vi "SetTemperatureSetPoint.vi"(2 "Temperature":sgl) -> ()   [LabVIEW 2011]
uses:
  GlobalVariables.vi
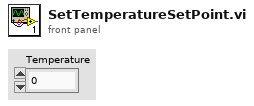
[diagram p1: front panel]
types:
  T1 = typedef "EZ-ZONE Output Cluster.ctl" = cluster{"Loop Control Mode":u32, "Closed Loop Set Point":sgl, "Open Loop Set Point":sgl, "Alarm 1 - High Set Point":sgl, "Alarm 1 - Low Set Point":sgl, "Alarm 2 - High Set Point":sgl, "Alarm 2 - Low Set Point":sgl, "Alarm 3 - High Set Point":sgl, "Alarm 3 - Low Set Point":sgl, "Alarm 4 - High Set Point":sgl, "Alarm 4 - Low Set Point":sgl, "Profile Action Request":u32, "Profile Start":u32, "Heat Proportional Band":sgl, "Cool Proportional Band":sgl, "Time Integral":sgl, "Time Derivative":sgl, "Heat Hysteresis":sgl, "Cool Hysteresis":sgl, "Dead Band":sgl}
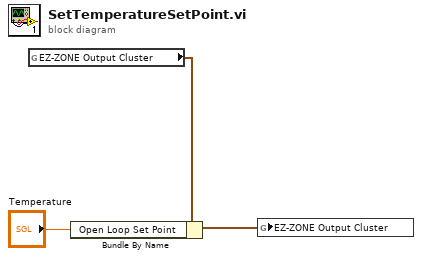
[diagram p0: block diagram]
diagram:
  n1 = global read "GlobalVariables.vi" "EZ-ZONE Output Cluster"() -> (w3:T1)
  n2 = Bundle By Name(cluster=w3, "Open Loop Set Point"="Temperature") -> (w2:T1)
  n3 = global write "GlobalVariables.vi" "EZ-ZONE Output Cluster"(w2) -> ()
